vi "Send_ShowDecoration.vi"(8 "error in":errorcluster, 9 "Visible":bool, 10 "index":i32, 11 "Queue in":refnum<queue>) -> (0 "error out":errorcluster)   [LabVIEW 2018, in "UI_Library.lvlib"]
uses:
  UI_Library.lvlib
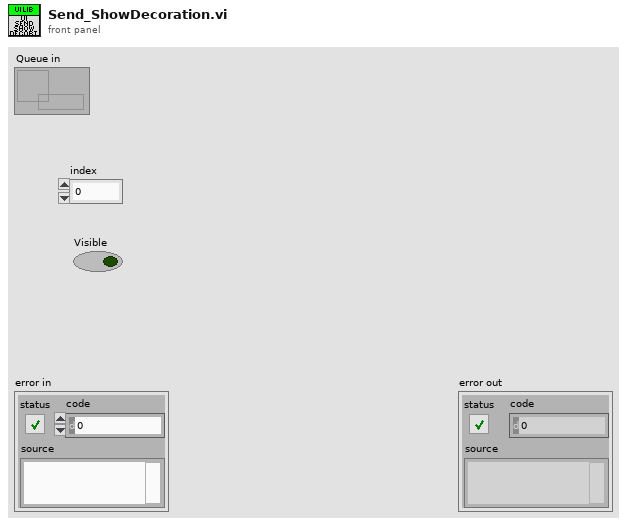
[diagram p1: front panel]
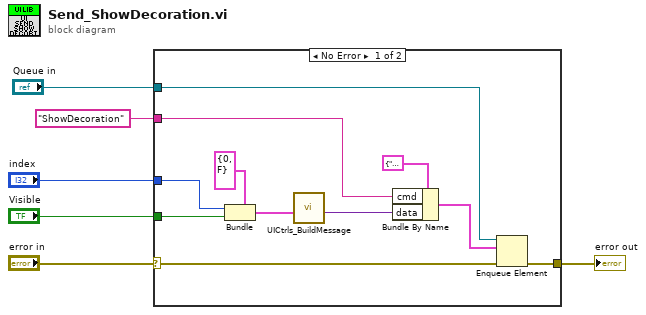
[diagram p0: block diagram]
diagram:
  n1 = case shown="No Error" "error in" {
    selector: "error in" -> [w16 w18]
    tunnel: "Queue in" -> [w17 _]
    tunnel: "ShowDecoration" ("UICmd") -> [w14 _]
    tunnel: [w15 w18] -> w6
    tunnel: "index" -> [w12 _]
    tunnel: "Visible" -> [w11 _]
    frame No Error {
      n2 = Bundle(cluster=cluster{"index":i32, "Visible":bool} {"index"=0, "Visible"=FALSE} ("Data"), "index"=w12, "Visible"=w11) -> (w10:cluster{"index":i32, "Visible":bool})
      n3 = call "UICtrls_BuildMessage.vi"("Control Data"=w10) -> ("Data"=w7:variant)  [unwired: 7 in]
      n4 = Bundle By Name(cluster=cluster{"cmd":string, "data":variant} {"cmd"="", "data"=variant} ("element"), "cmd"=w14, "data"=w7) -> (w8:cluster{"cmd":string, "data":variant})
      n5 = Enqueue Element(queue=w17, element=w8, error in (no error)=w16) -> (error out=w15:errorcluster)  [unwired: 1 in, 2 out]
    }
    frame Error {
    }
  }
  "error out" <- w6
